vi "Set_Parameters.vi"(8 "error in (no error)":errorcluster, 10 "Message_command In":T1, 11 "Command Queue In":T2) -> (0 "error out":errorcluster, 2 "Message_command Out":T1, 3 "Command Queue out":T2)   [LabVIEW 2020]
uses:
  Command_Queue.ctl
  Command_Message.ctl
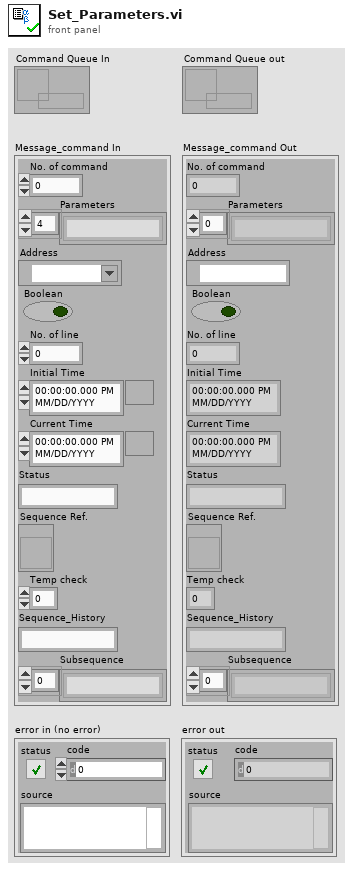
[diagram p1: front panel]
types:
  T1 = typedef "Command_Message.ctl" = cluster{"No. of command":i32, "Parameters":string[], "Address":refnum<visa-resource-name>, "Boolean":bool, "No. of line":i32, "Initial Time":timestamp, "Current Time":timestamp, "Status":string, "Sequence Ref.":refnum<vi>, "Temp check":i32, "Sequence_History":string, "Subsequence":string[]}
  T2 = typedef "Command_Queue.ctl" = refnum<queue>
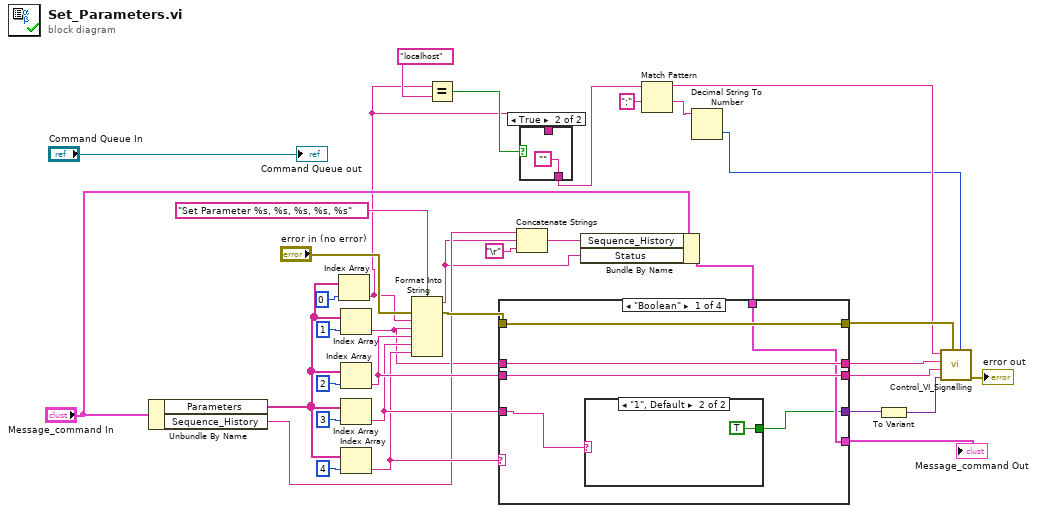
[diagram p0: block diagram]
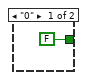
[diagram p3: hidden frame]
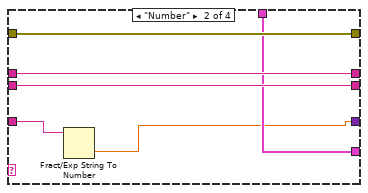
[diagram p4: hidden frame]
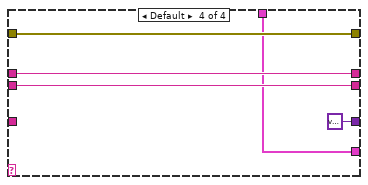
[diagram p6: hidden frame]
diagram:
  n1 = Unbundle By Name("Message_command In") -> ("Parameters"=w13:string[], "Sequence_History"=w20:string)
  n2 = Index Array(array=w13, index=0) -> (element=w3:string)
  n3 = Index Array(array=w13, index=1) -> (element=w11:string)
  n4 = Index Array(array=w13, index=2) -> (element=w29:string)
  n5 = Index Array(array=w13, index=3) -> (element=w28:string)
  n6 = Index Array(array=w13, index=4) -> (element=w27:string)
  n7 = Format Into String(format string="Set Parameter %s, %s, %s, %s, %s", error in="error in (no error)", w3, w11, w29, w28, w27) -> (resulting string=w17:string, error out=w26:errorcluster)  [unwired: 1 in]
  n8 = Equal?(x=w3, y="localhost") -> (x = y?=w9:bool)
  n9 = Concatenate Strings(w20, w17, "\r") -> (w18:string)
  n10 = case shown="True" w9 {
    tunnel: [w36 ""] -> w6
    tunnel: w3 -> [w36 _]
    frame False {
    }
    frame True {
    }
  }
  n11 = Bundle By Name(cluster="Message_command In", "Sequence_History"=w18, "Status"=w17) -> (w16:T1)
  n12 = case shown="\"Boolean\"" w27 {
    tunnel: w11 -> [w43 w50 w55 w60]
    tunnel: w29 -> [w42 w49 w54 w59]
    tunnel: [w43 w50 w55 w60] -> w24
    tunnel: [w42 w49 w54 w59] -> w23
    tunnel: w28 -> [w39 w47 w52 _]
    tunnel: [w38 w46 w52 variant ("Variant")] -> w1
    tunnel: w26 -> [w41 w51 w56 w61]
    tunnel: [w41 w51 w56 w61] -> w25
    tunnel: [w40 w48 w53 w57] -> w15
    tunnel: w16 -> [w40 w48 w53 w57]
    frame "Boolean" {
      n13 = case shown="\"1\", Default" w39 {
        tunnel: [FALSE TRUE] -> w38
        frame "0" {
        }
        frame "1", Default {
        }
      }
    }
    frame "Number" {
      n14 = Fract/Exp String To Number(string=w47) -> (number=w46:dbl)  [unwired: 3 in, 1 out]
    }
    frame "String" {
    }
    frame Default {
    }
  }
  "Message_command Out" <- w15
  n15 = Match Pattern(string=w6, regular expression=":") -> (before substring=w5:string, after substring=w7:string)  [unwired: 1 in, 2 out]
  n16 = Decimal String To Number(string=w7) -> (number=w4:i32)  [unwired: 2 in, 1 out]
  n17 = To Variant(anything=w1) -> (Variant=w2:variant)
  n18 = call "Control_VI_Signalling.vi"("port number"=w4, "error in (no error)"=w25, "Input Value"=w2, "Control Name"=w23, "Target VI name"=w24, "Machine Name"=w5) -> ("error out"=→"error out":errorcluster)  [unwired: 5 in]
  "Command Queue out" <- "Command Queue In"
